vi "Write Abort Notifier 2.vi"(8 "error in (no error)":errorcluster, 10 "Abort Notifier":refnum<notifier>, 11 "AFM_Driver in":refnum<class "AFM_Driver.lvclass">) -> (0 "error out":errorcluster, 3 "AFM_Driver out":refnum<class "AFM_Driver.lvclass">)   [LabVIEW 2019, in "AFM_Driver.lvclass"]
uses:
  AFM_Driver.lvclass
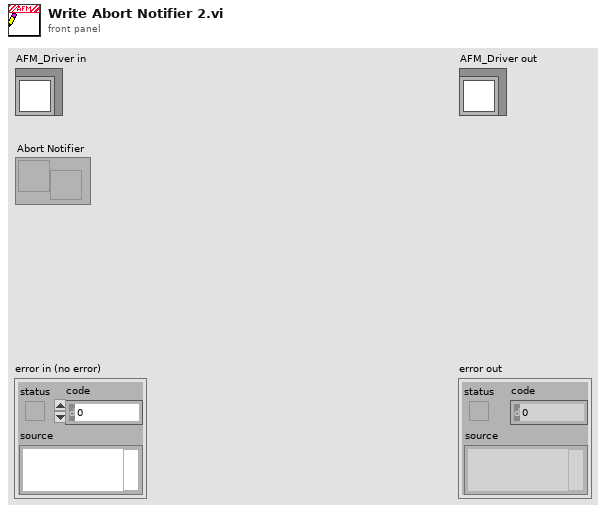
[diagram p1: front panel]
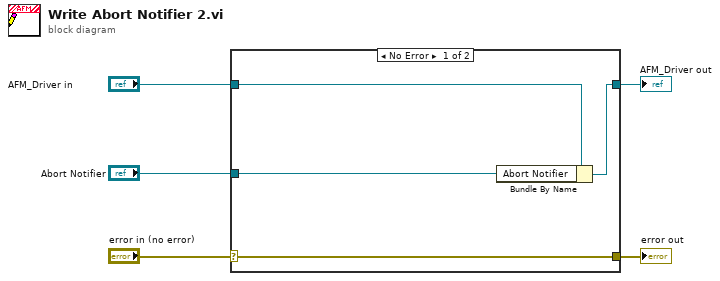
[diagram p0: block diagram]
diagram:
  n1 = case shown="No Error" "error in (no error)" {
    selector: "error in (no error)" -> [w9 w10]
    tunnel: [w9 w10] -> w4
    tunnel: [w7 w11] -> w2
    tunnel: "AFM_Driver in" -> [w8 w11]
    tunnel: "Abort Notifier" -> [w6 _]
    frame No Error {
      n2 = Bundle By Name(cluster=w8, "Abort Notifier"=w6) -> (w7:refnum<class "AFM_Driver.lvclass">)
    }
    frame Error {
    }
  }
  "error out" <- w4
  "AFM_Driver out" <- w2
